vi "Rx IPv4 Frame Payload to data.vi"(7 "Payload array":u8[](array[numeric])) -> (4 "Source IP":u8[](array[numeric]), 6 "Destination Port":u16, 8 "Source Port":u16, 10 "Protocol":T1, 15 "RF data":string)   [LabVIEW 2014]
uses:
  Protocol enum.ctl
  a0cb46ee-4e19-4156-9b2b-388afd7d0907.vi
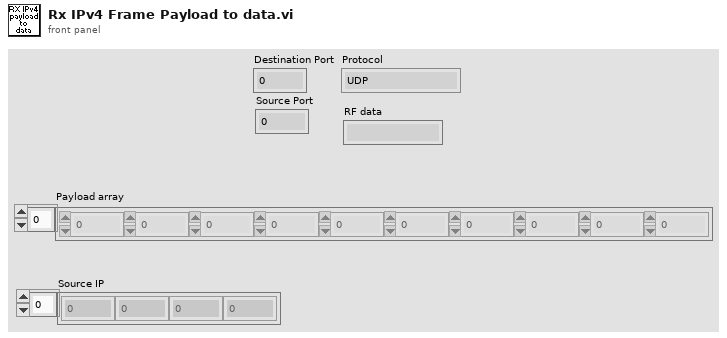
[diagram p1: front panel]
types:
  T1 = typedef "Protocol enum.ctl" = enum8{"UDP", "TCP"}
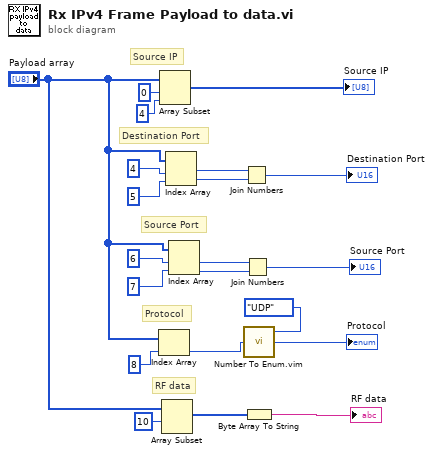
[diagram p0: block diagram]
diagram:
  # "RF data"
  # "Protocol"
  # "Source Port"
  # "Destination Port"
  # "Source IP"
  n1 = Index Array(array="Payload array", index=8) -> (element=w6:u8)
  n2 = Array Subset(array="Payload array", index=0, length=4) -> (→"Source IP":u8[])
  n3 = Array Subset(array="Payload array", index=10) -> (w3:u8[])  [unwired: 1 in]
  n4 = Index Array(array="Payload array", index #1=4 ("index"), index #2=5 ("index")) -> (element #1=w12:u8, element #2=w11:u8)
  n5 = Index Array(array="Payload array", index #1=6 ("index"), index #2=7 ("index")) -> (element #1=w10:u8, element #2=w9:u8)
  n6 = Join Numbers(hi=w12, lo=w11) -> ((hi.lo)=→"Destination Port":u16)
  n7 = Join Numbers(hi=w10, lo=w9) -> ((hi.lo)=→"Source Port":u16)
  n8 = call "Number To Enum.vim"("number"=w6, "enum type"=Protocol_enum."UDP") -> ("number as enum"=→"Protocol":T1)
  n9 = Byte Array To String(unsigned byte array=w3) -> (string=→"RF data":string)
